vi "ArrayToTags.vi"(1 "Array":string[](array[string])) -> (0 "String":string)   [LabVIEW 2013]
doc: "Converts array of XML tags to a string. Appends each tag to the one before it"
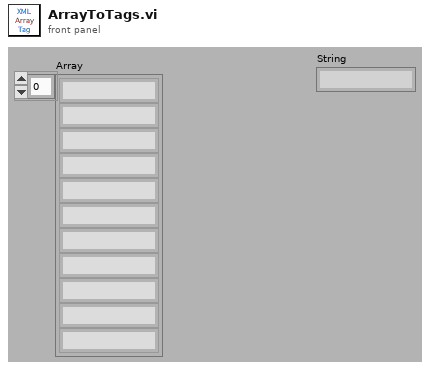
[diagram p1: front panel]
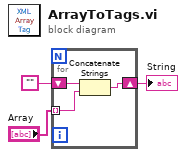
[diagram p0: block diagram]
diagram:
  n1 = for {
    tunnel: "Array" -> [w4] mode=indexing
    shift-right: [w5] -> w1
    shift-left: "" -> [w6]
    n2 = Concatenate Strings(w6, w4) -> (w5:string)
  }
  "String" <- w1
